vi "DIOSerialPort.vi"(10 "DIOSerialPortSettings":T1={"TxPort"="GyroSubnetTx", "TxDataFIFO"="GyroTxDataFIFO", "TxHealthAndStatusFIFO"="GyroTxHealthAndStatusFIFO", "RxPort"="GyroSubnetRx", "RxDataFIFO"="GyroRxDataFIFO", "RxHealthAndStatusFIFO"="GyroRxHealthAndStatusFIFO", "BaseHealthAndStatusAddress"=0, "TimestampRegister"="TimestampRegister", "TxTimestampFIFO"="GyroTxTimestampFIFO"}) -> ()   [LabVIEW 2016, in "FPGADIOSerialASCII.lvlib"]
uses:
  FPGADIOSerialASCII.lvlib
  DataTypes/DIOSerialPortSettings.ctl
  <vilib>/rvi/eio/common/nirviEmuTemplateMethod_errors.vi
  <vilib>/rvi/Emulation/niFpgaProcessEmulError.vi
  <vilib>/eio/EIONode/EIONode.xnode
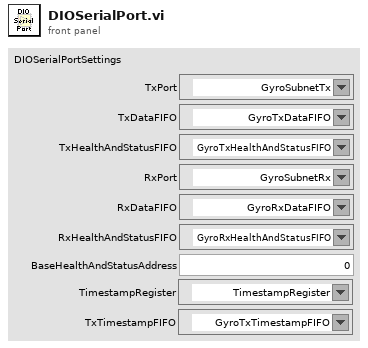
[diagram p1: front panel]
types:
  T1 = typedef "FPGADIOSerialASCII.lvlib/DIOSerialPortSettings.ctl" = cluster{"TxPort":refnum<k21>, "TxDataFIFO":refnum<k21>, "TxHealthAndStatusFIFO":refnum<k21>, "RxPort":refnum<k21>, "RxDataFIFO":refnum<k21>, "RxHealthAndStatusFIFO":refnum<k21>, "BaseHealthAndStatusAddress":u32, "TimestampRegister":refnum<k21>, "TxTimestampFIFO":refnum<k21>}
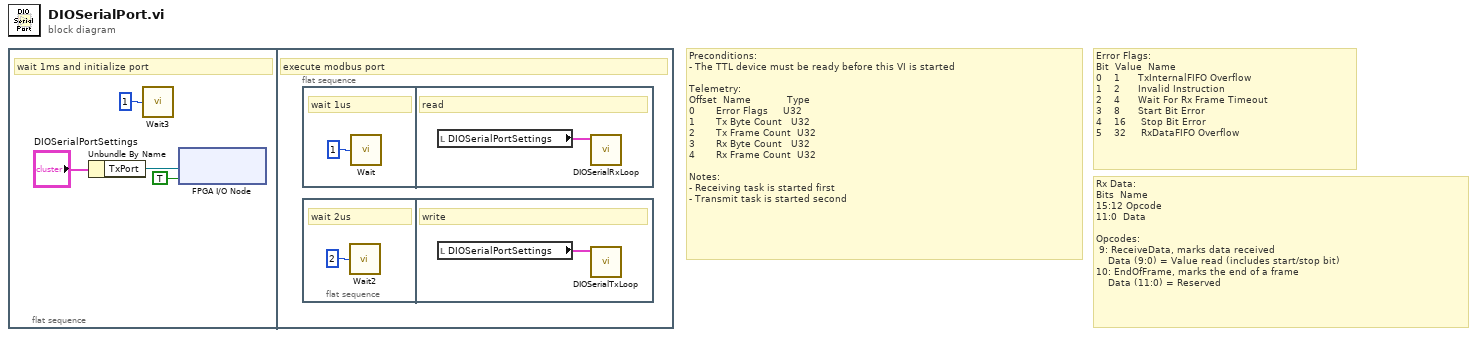
[diagram p0: block diagram]
diagram:
  # "Rx Data:\nBits  Name\n15:12 Opcode\n11:0  Data\n\nOpcodes:\n 9: ReceiveData, marks data received\n    Data (9:0) = Value read (includes start/stop bit)\n10: EndOfFrame, marks the end of a frame\n    Data (11:0) = Reserved"
  # "Error Flags:\nBit  Value  Name\n0    1      TxInternalFIFO Overflow\n1    2      Invalid Instruction \n2    4      Wait For Rx Frame Timeout\n3    8      Start Bit Error\n4    16     Stop Bit Error\n5    32     RxDataFIFO Overflow"
  # "Preconditions:\n- The TTL device must be ready before this VI is started\n\nTelemetry:\nOffset  Name            Type\n0       Error Flags     U32         \n1       Tx Byte Count   U32\n2       Tx Frame Count  U32\n3       Rx Byte Count   U32\n4       Rx Frame Count  U32\n\nNotes:\n- Receiving task is started first\n- Transmit task is started second"
  n1 = flat-sequence {
    frame #0 {
      # "wait 1ms and initialize port"
      n2 = Unbundle By Name("DIOSerialPortSettings") -> ("TxPort"=w2:refnum<k21>)
      n3 = call "Wait3"("Count(mSec)"=u32 1 ("Count(Ticks)")) -> ()  [unwired: 1 out]
      n4 = xnode "FPGA I/O Node"("I/O Item"=TRUE, "FPGA I/O In"=w2) -> ()  [unwired: 1 out]
    }
    frame #1 {
      # "execute modbus port"
      n5 = flat-sequence {
        frame #0 {
          # "wait 1us"
          n6 = call "Wait"("Count(uSec)"=u32 1 ("Count(Ticks)")) -> ()  [unwired: 1 out]
        }
        frame #1 {
          # "read"
          n7 = local read "DIOSerialPortSettings"() -> (w8:T1)
          n8 = call "DIOSerialRxLoop.vi"("DIOSerialPortSettings"=w8) -> ()  [unwired: 11 in]
        }
      }
      n9 = flat-sequence {
        frame #0 {
          # "wait 2us"
          n10 = call "Wait2"("Count(uSec)"=u32 2 ("Count(Ticks)")) -> ()  [unwired: 1 out]
        }
        frame #1 {
          # "write"
          n11 = local read "DIOSerialPortSettings"() -> (w6:T1)
          n12 = call "DIOSerialTxLoop.vi"("DIOSerialPortSettings"=w6) -> ()  [unwired: 11 in]
        }
      }
    }
  }
